vi "Clust Get ClassID.vi"(11 "Ctl Refnum":refnum<vi>) -> (3 "ClassID":T1)   [LabVIEW 2014]
uses:
  Clust ClassID.ctl
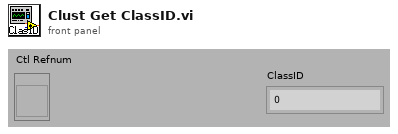
[diagram p1: front panel]
types:
  T1 = typedef "Clust ClassID.ctl" = enum16{"０", "１", "２", "３", "４", "５", "６", "色", "ブール", "９", "１０", "パス", "１２", "１３", "配列", "１５", "１６", "１７", "数値", "１９", "２０", "２１", "２２", "２３", "２４", "２５", "２６", "文字列", "２８", "２９", "３０", "３１", "３２", "３３", "リング", "Enum", "３６"}
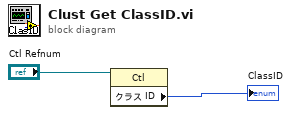
[diagram p0: block diagram]
diagram:
  n1 = property class="Ctl"(reference="Ctl Refnum") -> ("クラス ID"=→"ClassID":u32)  [unwired: 1 in, 2 out]
